vi "VIS-IR_INIT_brd.vi"(1 "AdrDelay":u32=4096 format="%.0x", 2 "pclk":u32=2 format="%.0x", 4 "PPortAddress":u32=888 format="%.0x", 5 "flag816":u32=2, 6 "waits":u32, 7 "pixel":u32=5400, 8 "error in (no error)":errorcluster, 9 "burst":u8, 10 "sym":u8=1, 11 "VIS-IR in":refnum<class "VIS-NIR.lvclass">) -> (0 "error out":errorcluster, 3 "VIS-IR out":refnum<class "VIS-NIR.lvclass">)   [LabVIEW 2015, in "VIS-NIR.lvclass"]
uses:
  VIS-NIR.lvclass
  Detector.lvclass/Detector.ctl
  Detector.lvclass
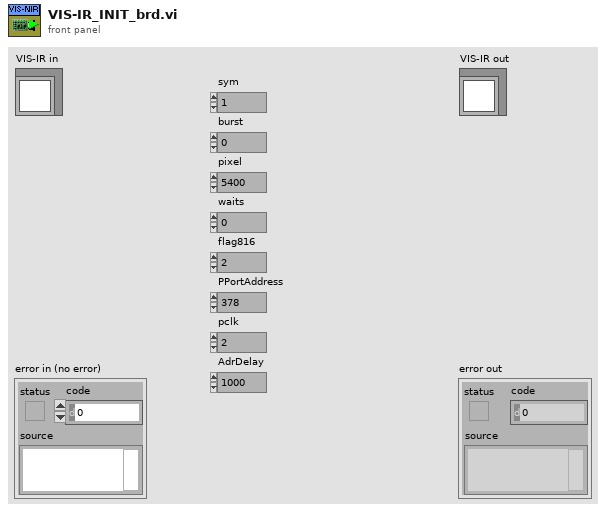
[diagram p1: front panel]
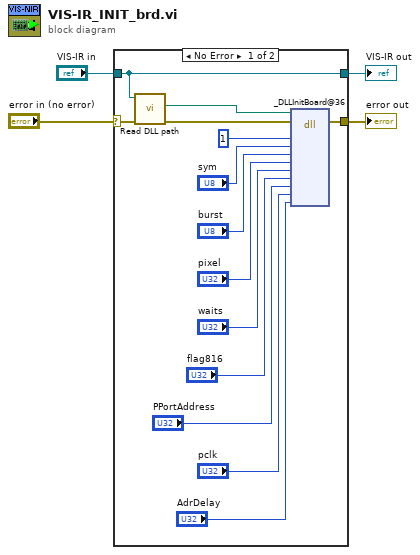
[diagram p0: block diagram]
diagram:
  n1 = case shown="No Error" "error in (no error)" {
    selector: "error in (no error)" -> [w17 w20]
    tunnel: [w6 w20] -> w3
    tunnel: [w18 w19] -> w1
    tunnel: "VIS-IR in" -> [w18 w19]
    frame No Error {
      n2 = call "Read DLL path.vi"("error in (no error)"=w17, "Detector in"=w18) -> ("error out"=w7:errorcluster, "DLL path"=w5:path)  [unwired: 7 in, 1 out]
      n3 = dll-call lib="G:/SD/TRANCON/DLL/ESLSCDLL.dll" fn="_DLLInitBoard@36"(path in=w5, error in=w7, "drv"=u32 1, "sym"="sym", "burst"="burst", "pixel"="pixel", "waits"="waits", "flag816"="flag816", "pportadr"="PPortAddress", "pclk"="pclk", "xckdelay"="AdrDelay") -> (error out=w6:errorcluster)  [unwired: 11 in, 1 out]
    }
    frame Error {
    }
  }
  "error out" <- w3
  "VIS-IR out" <- w1
